vi "Tree.vi"   [LabVIEW 2020, in "NI_DataFinder.lvlib"]
doc: "Contains an overview of all the DataFinder VIs."
uses:
  <vilib>/DataFinder/NI_DataFinder.lvlib
  <vilib>/DataFinder/Get Property Values (String Property).vi
  <vilib>/DataFinder/Create Query (String).vi
  <vilib>/DataFinder/Close Reference (DataFinder).vi
  <vilib>/DataFinder/Results to Waveforms (ddt).vi
  <vilib>/DataFinder/Get Indexed Value Limits (Numeric).vi
  <vilib>/userdefined/High Color/DFDataFinder.ctl
  <vilib>/userdefined/NI_DataFinder Controls.lvlib
panel:
  # "Open block diagram to view the DataFinder Toolkit VI tree."
types:
  T1 = typedef "NI_DataFinder Controls.lvlib/DFDataFinder.ctl" = refnum<k21>
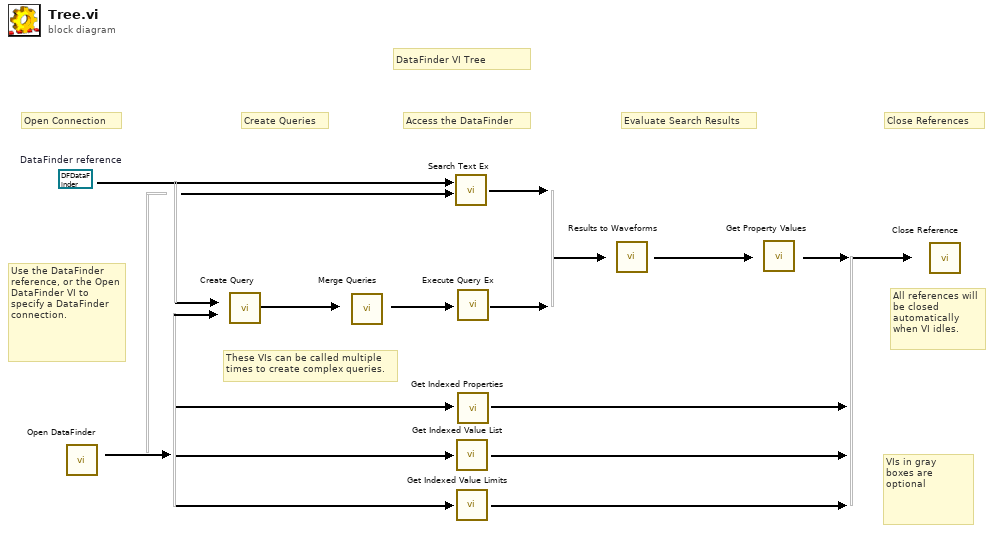
[diagram p0: block diagram]
diagram:
  (unwired) T1 refnum  # DataFinder reference
  # "Access the DataFinder"
  # "Use the DataFinder reference, or the Open DataFinder VI to specify a DataFinder connection."
  # "All references will be closed\nautomatically when VI idles."
  # "DataFinder VI Tree"
  # "VIs in gray\nboxes are\noptional"
  # "These VIs can be called multiple\ntimes to create complex queries."
  # "Create Queries"
  # "Evaluate Search Results"
  # "Close References"
  # "Open Connection"
  n1 = call <vilib>:"Open DataFinder.vi"() -> ()  [unwired: 14 in, 2 out]
  n2 = call-poly <vilib>:"Create Query.vi"() -> ()  [unwired: 14 in, 2 out]
  n3 = call <vilib>:"Merge Queries.vi"() -> ()  [unwired: 14 in, 2 out]
  n4 = call <vilib>:"Search Text Ex.vi"() -> ()  [unwired: 11 in, 5 out]
  n5 = call <vilib>:"Get Indexed Value List.vi"() -> ()  [unwired: 11 in, 5 out]
  n6 = call-poly <vilib>:"Get Indexed Value Limits.vi"() -> ()  [unwired: 11 in, 5 out]
  n7 = call <vilib>:"Execute Query Ex.vi"() -> ()  [unwired: 10 in, 6 out]
  n8 = call <vilib>:"Get Indexed Properties.vi"() -> ()  [unwired: 13 in, 3 out]
  n9 = call-poly <vilib>:"Results to Waveforms.vi"() -> ()  [unwired: 13 in, 3 out]
  n10 = call-poly <vilib>:"Get Property Values.vi"() -> ()  [unwired: 13 in, 3 out]
  n11 = call-poly <vilib>:"Close Reference.vi"() -> ()  [unwired: 15 in, 1 out]
